vi "MListbox Move Selected Down.vi"(8 "error in (no error)":errorcluster, 11 "Multicolumn ListBox in":refnum<class "Multicolumn ListBox.lvclass">) -> (0 "error out":errorcluster, 3 "Multicolumn ListBox out":refnum<class "Multicolumn ListBox.lvclass">)   [LabVIEW 2012, in "Multicolumn ListBox.lvclass"]
uses:
  Multicolumn ListBox.lvclass
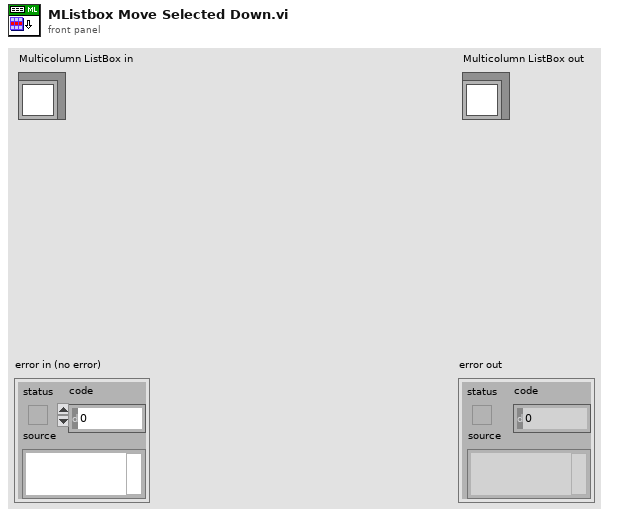
[diagram p1: front panel]
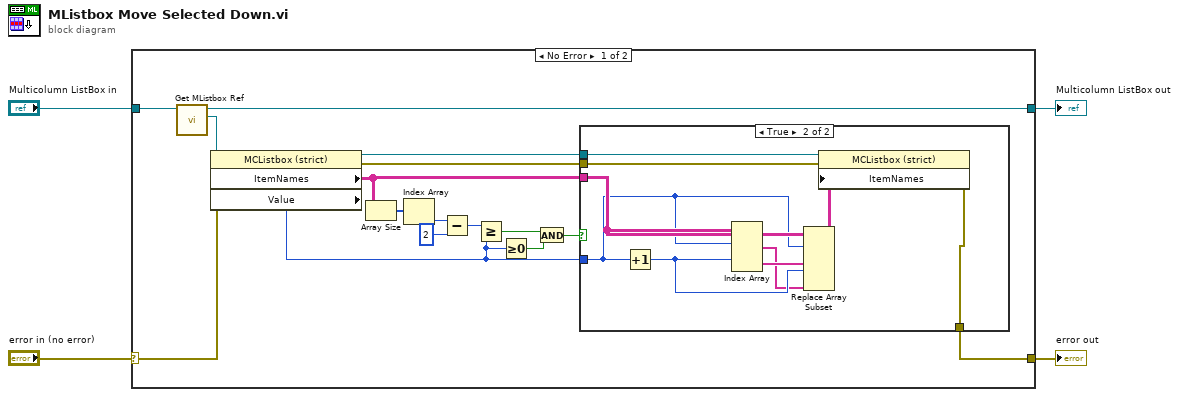
[diagram p0: block diagram]
diagram:
  n1 = case shown="No Error" "error in (no error)" {
    selector: "error in (no error)" -> [w15 w32]
    tunnel: [w14 w32] -> w3
    tunnel: [w19 w31] -> w1
    tunnel: "Multicolumn ListBox in" -> [w20 w31]
    frame No Error {
      n2 = call "Get MListbox Ref.vi"("Multicolumn ListBox in"=w20) -> ("MListbox Ref"=w18:refnum<vi>, "Multicolumn ListBox out"=w19:refnum<class "Multicolumn ListBox.lvclass">)  [unwired: 8 in, 1 out]
      n3 = property class="MCListbox (strict)"(reference=w18, error in=w15) -> (reference out=w17:refnum<vi>, error out=w16:errorcluster, "ItemNames"=w13:string[][], "Value"=w6:i32)
      n4 = Array Size(array=w13) -> (size(s)=w12:i32[])
      n5 = Index Array(array=w12) -> (element=w11:i32)  [unwired: 1 in]
      n6 = Subtract(x=w11, y=2) -> (x-y=w9:i32)
      n7 = Greater Or Equal?(x=w9, y=w6) -> (x >= y?=w8:bool)
      n8 = Greater Or Equal To 0?(x=w6) -> (x >= 0?=w5:bool)
      n9 = And(x=w8, y=w5) -> (x .and. y?=w7:bool)
      n10 = case shown="True" w7 {
        tunnel: w17 -> [_ w30]
        tunnel: w16 -> [w21 w29]
        tunnel: [w21 w28] -> w14
        tunnel: w13 -> [_ w27]
        tunnel: w6 -> [_ w22]
        frame False {
        }
        frame True {
          n11 = Increment(x=w22) -> (x+1=w25:i32)
          n12 = Index Array(array=w27, index (row) #1=w22, index (row) #2=w25) -> (element #1=w24:string[], element #2=w26:string[])  [unwired: 2 in]
          n13 = Replace Array Subset(array=w27, new element #1=w26, index (row) #1=w22, new element #2=w24, index (row) #2=w25) -> (w23:string[][])  [unwired: 2 in]
          n14 = property class="MCListbox (strict)"(reference=w30, error in=w29, "ItemNames"=w23) -> (error out=w28:errorcluster)  [unwired: 1 out]
        }
      }
    }
    frame Error {
    }
  }
  "error out" <- w3
  "Multicolumn ListBox out" <- w1
